vi "Delete Class Reference.vi"(8 "error in (no error)":errorcluster, 11 "ParentClass in":refnum<class "ParentClass.lvclass">) -> (0 "error out":errorcluster, 3 "ParentClass out":refnum<class "ParentClass.lvclass">)   [LabVIEW 2012, in "ParentClass.lvclass"]
uses:
  ParentClass.lvclass
  ParentClass.lvclass/ParentClass.ctl
panel:
  in  "Class Reference":refnum<data-value>
  # "Method is not used.\n\nThis method of constructing\nreferences does not work like I\nhad planned.\n\nTry it yourself to see what goes wrong!"
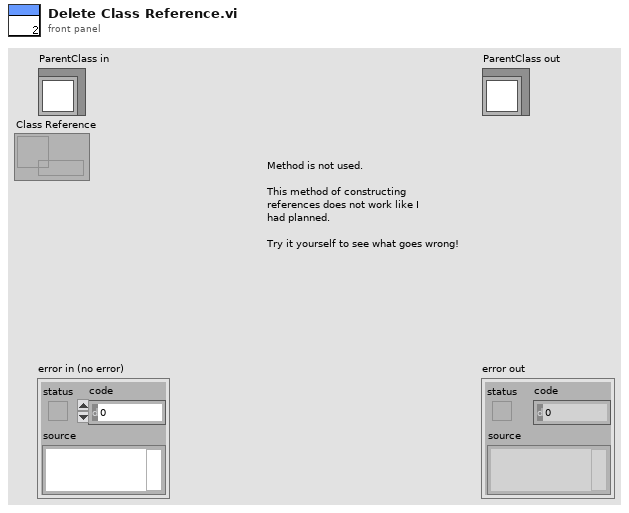
[diagram p1: front panel]
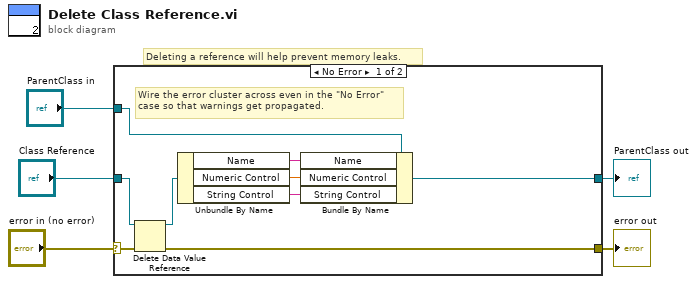
[diagram p0: block diagram]
diagram:
  # "Deleting a reference will help prevent memory leaks."
  n1 = case shown="No Error" "error in (no error)" {
    selector: "error in (no error)" -> [w13 w16]
    tunnel: [w12 w16] -> w4
    tunnel: [w6 w15] -> w2
    tunnel: "ParentClass in" -> [w10 w15]
    tunnel: "Class Reference" -> [w14 _]
    frame No Error {
      # "Wire the error cluster across even in the \"No Error\"\ncase so that warnings get propagated."
      n2 = Delete Data Value Reference(data value reference=w14, error in=w13) -> (data value=w11:refnum<class "ParentClass.lvclass">, error out=w12:errorcluster)
      n3 = Unbundle By Name(w11) -> ("Name"=w9:string, "Numeric Control"=w8:dbl, "String Control"=w7:string)
      n4 = Bundle By Name(cluster=w10, "Name"=w9, "Numeric Control"=w8, "String Control"=w7) -> (w6:refnum<class "ParentClass.lvclass">)
    }
    frame Error {
    }
  }
  "error out" <- w4
  "ParentClass out" <- w2
